vi "Controller Error Handling Loop.vi"(7 "Sync Objects":T1, 8 "error in (no error)":errorcluster, 11 "FOFB Configuration":T4={"FOFB Parameters"={"Network"={"FOFB Controller IP"="", "LNLS Control Network IP"="", "LNLS Control Network Power Supplies TCP Port"=0, "LNLS Control Network FOFB Configuration TCP Port"=0, "LNLS Control Network BPMs TCP Port"=0, "Monitoring Data TCP Port"=0, "Fast Archiver TCP Port"=0, "Fast Command TCP Port"=0, "TCP Listening Timeout"=0}, "Fast Acquisition"={"Sampling Period"=0, "Data Buffer Size"=0, "Monitoring Period"=0}, "Acquisition Network"=[], "Actuation Network"=[]}, "Number of Acquisition Chassis"=0, "Number of Actuation Chassis"=0, "Number of BPM Readings"=0, "BPM Reading Names"=[], "Selected BPM Readings"=[0, 1, 2, 3, 4, 5, 6, 7, 8, 9, 10, 11, 12, 13, 14, 15, 16, 17, 18, 19, 20, 21, 22, 23, 24, 25, 26, 27, 28, 29, 30, 31, 32, 33, 34, 35, 36, 37, 38, 39, 40, 41, 42, 43, 44, 45, 46, 47, 48, 49], "Number of Correctors"=0, "Corrector Names"=[], "Selected Correctors"=[0, 1, 2, 3, 4, 5, 6, 7, 8, 9, 10, 11, 12, 13, 14, 15, 16, 17, 18, 19, 20, 21, 22, 23, 24, 25, 26, 27, 28, 29, 30, 31, 32, 33, 34, 35, 36, 37, 38, 39, 40, 41, 42, 43, 44, 45, 46, 47, 48, 49], "Response Matrix"=[], "Reference Orbit"=[], "Correction Matrix"=[], "FPGA Filter Sets"=[], "Acquisition Chassis Names"=[], "Actuation Chassis Names"=[], "Acquisition Variables"=[], "Actuation Variables"=[], "PS Matrix Mapping"=[], "Inverse PS Matrix Mapping"=[], "BPM Matrix Mapping"=[], "Inverse BPM Matrix Mapping"=[], "BPM Planes"=[], "Corrector Planes"=[]}) -> (0 "error out":errorcluster)   [LabVIEW 2011, in "Controller VIs.lvlib"]
uses:
  Controller VIs.lvlib
  Types Definitions/Type FOFB Configuration.ctl
  Types Definitions/Type FOFB Parameters.ctl
  Types Definitions/Type Network Configuration.ctl
  Types Definitions/Type FA Configuration.ctl
  Types Definitions/Type Acquisition Network Configuration.ctl
  Types Definitions/Type Actuation Network Configuration.ctl
  Types Definitions/Type Synchronization Objects.ctl
  Types Definitions/Type Blocking Synchronization Objects.ctl
  Types Definitions/Type Monitoring Data.ctl
  Types Definitions/Type Operation Mode State.ctl
  Types Definitions/Type Diagnostics Data.ctl
  Types Definitions/Type CPU Loads Array.ctl
  Types Definitions/Type CPU Loads.ctl
  Types Definitions/Type Non-blocking Synchronization Objects.ctl
  Types Definitions/Type FOFB Variables.ctl
  Types Definitions/Type Actuation State.ctl
  <vilib>/Platform/TimedLoop/XDataNode/timing_clust.ctl
  <vilib>/Platform/TimedLoop/XDataNode/nitl_modes.ctl
  <vilib>/Platform/TimedLoop/XDataNode/wakeup.ctl
  <vilib>/Platform/TimedLoop/XDataNode/XDataNode.xnode
  <vilib>/Platform/TimedLoop/XDataNode/XDNodeRunTimeDep.lvlib
  Type Definitions.lvlib
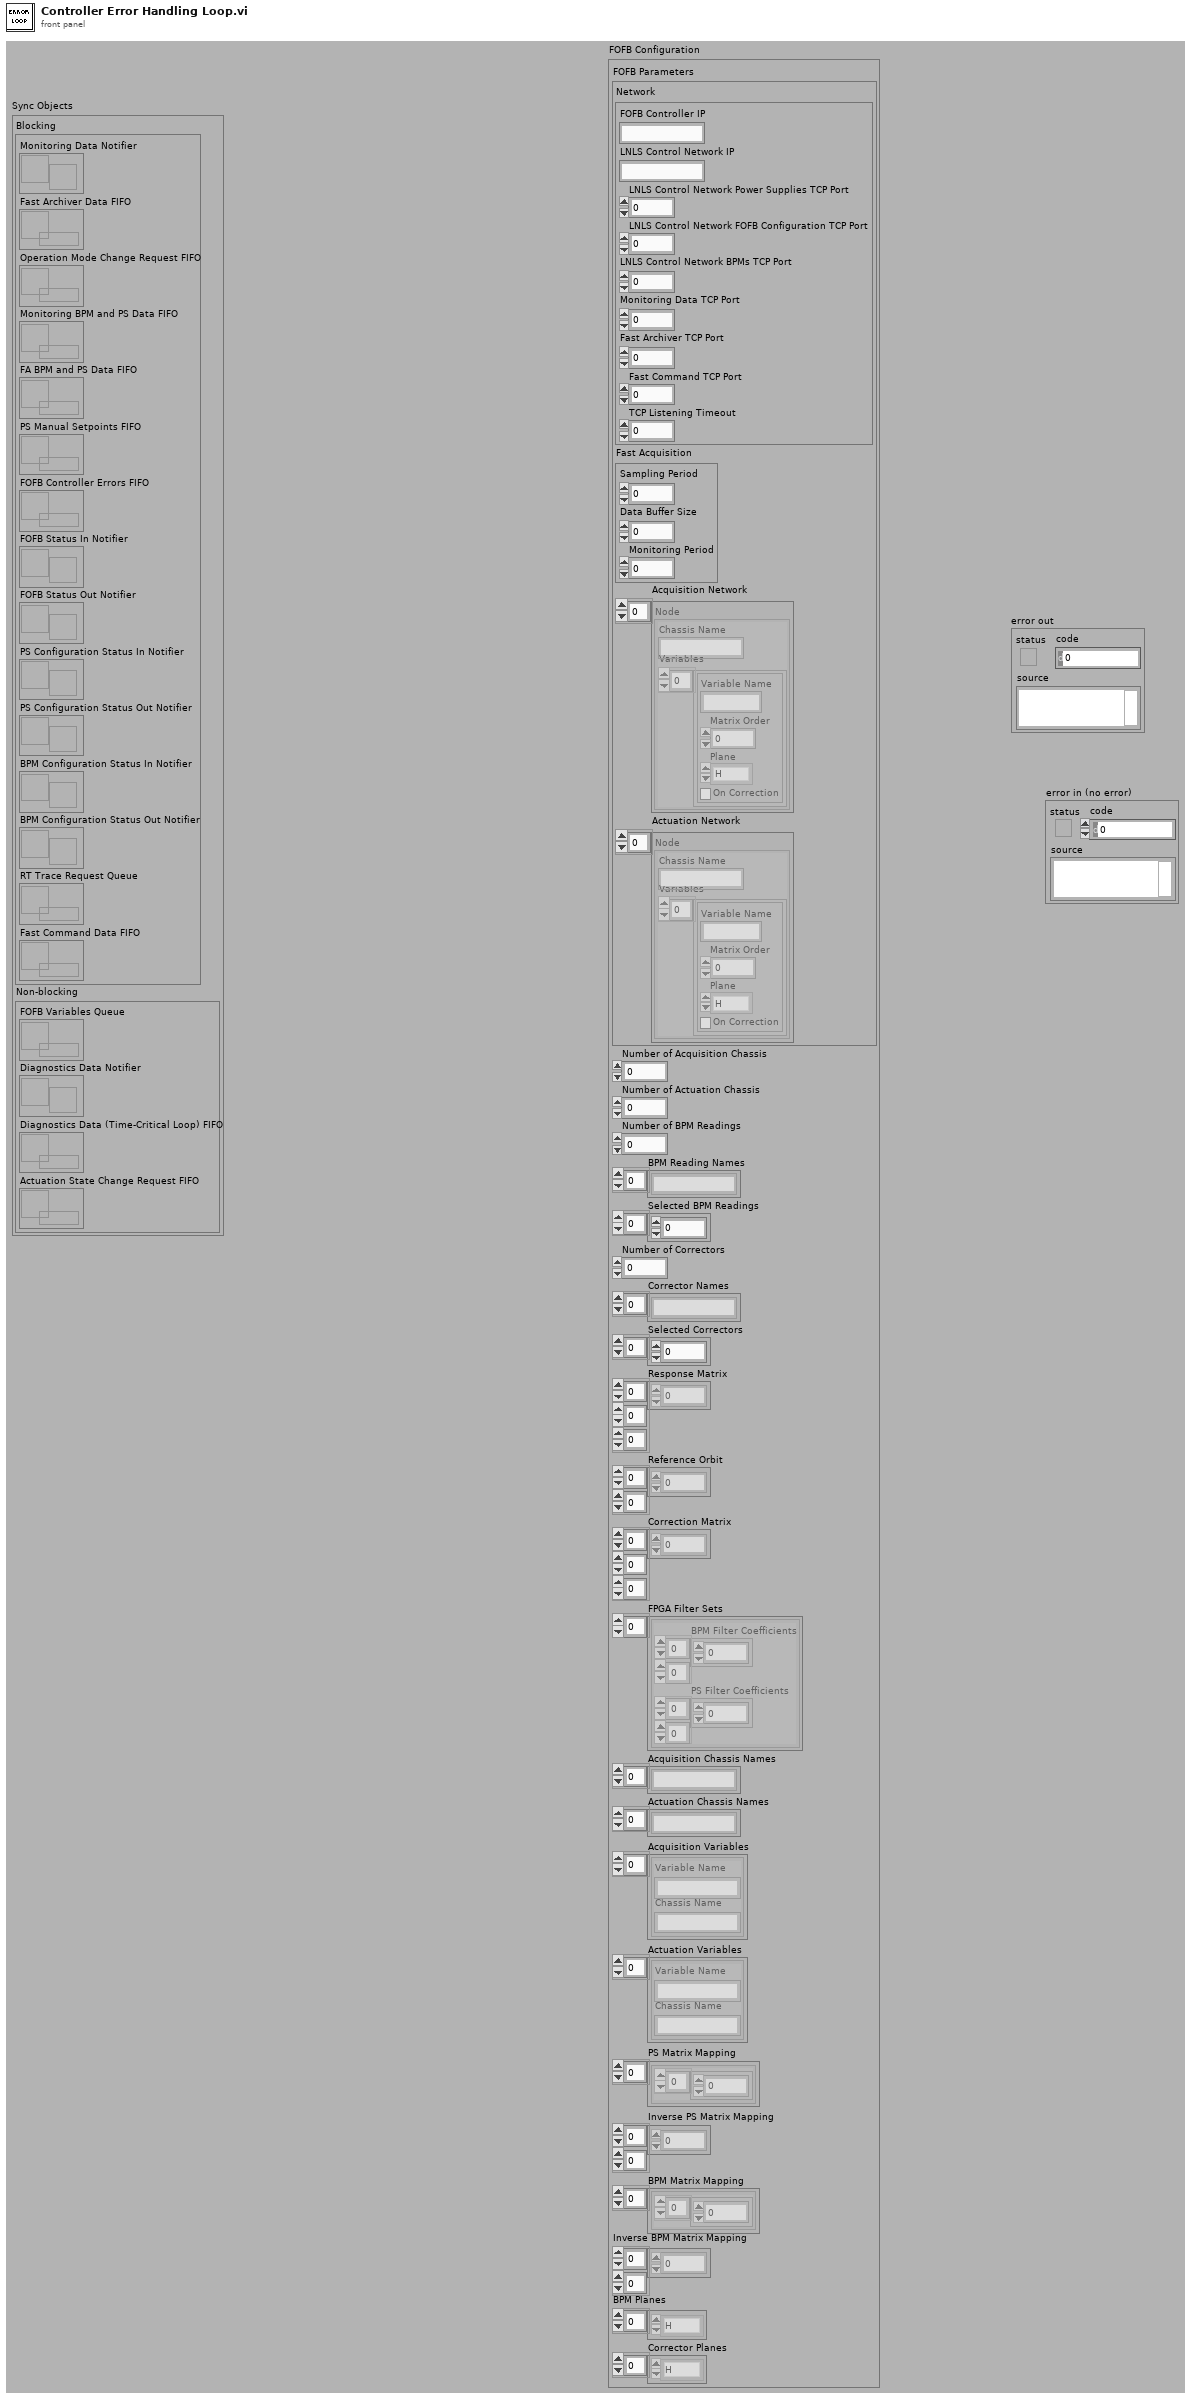
[diagram p1: front panel]
types:
  T1 = typedef "Type Definitions.lvlib/Type Synchronization Objects.ctl" = cluster{"Blocking":T2, "Non-blocking":T3}
  T2 = typedef "Type Definitions.lvlib/Type Blocking Synchronization Objects.ctl" = cluster{"Monitoring Data Notifier":refnum<notifier>, "Fast Archiver Data FIFO":refnum<queue>, "Operation Mode Change Request FIFO":refnum<k33>, "Monitoring BPM and PS Data FIFO":refnum<k33>, "FA BPM and PS Data FIFO":refnum<k33>, "PS Manual Setpoints FIFO":refnum<k33>, "FOFB Controller Errors FIFO ":refnum<k33>, "FOFB Status In Notifier":refnum<notifier>, "FOFB Status Out Notifier":refnum<notifier>, "PS Configuration Status In Notifier":refnum<notifier>, "PS Configuration Status Out Notifier":refnum<notifier>, "BPM Configuration Status In Notifier":refnum<notifier>, "BPM Configuration Status Out Notifier":refnum<notifier>, "RT Trace Request Queue":refnum<queue>, "Fast Command Data FIFO":refnum<k33>}
  T3 = typedef "Type Definitions.lvlib/Type Non-blocking Synchronization Objects.ctl" = cluster{"FOFB Variables Queue":refnum<queue>, "Diagnostics Data Notifier":refnum<notifier>, "Diagnostics Data (Time-Critical Loop) FIFO":refnum<k33>, "Actuation State Change Request FIFO":refnum<k33>}
  T4 = typedef "Type Definitions.lvlib/Type FOFB Configuration.ctl" = cluster{"FOFB Parameters":T5, "Number of Acquisition Chassis":i32, "Number of Actuation Chassis":i32, "Number of BPM Readings":i32, "BPM Reading Names":string[], "Selected BPM Readings":u32[], "Number of Correctors":i32, "Corrector Names":string[], "Selected Correctors":u32[], "Response Matrix":dbl[][][], "Reference Orbit":dbl[][], "Correction Matrix":dbl[][][], "FPGA Filter Sets":cluster{"BPM Filter Coefficients":dbl[][], "PS Filter Coefficients":dbl[][]}[], "Acquisition Chassis Names":string[], "Actuation Chassis Names":string[], "Acquisition Variables":cluster{"Variable Name":string, "Chassis Name":string}[], "Actuation Variables":cluster{"Variable Name":string, "Chassis Name":string}[], "PS Matrix Mapping":cluster{u32[]}[], "Inverse PS Matrix Mapping":u32[][], "BPM Matrix Mapping":cluster{u32[]}[], "Inverse BPM Matrix Mapping":u32[][], "BPM Planes":enum8{"H", "V"}[], "Corrector Planes":enum8{"H", "V"}[]}
  T5 = typedef "Type Definitions.lvlib/Type FOFB Parameters.ctl" = cluster{"Network":T6, "Fast Acquisition":T7, "Acquisition Network":T8, "Actuation Network":T9}
  T6 = typedef "Type Definitions.lvlib/Type Network Configuration.ctl" = cluster{"FOFB Controller IP":string, "LNLS Control Network IP":string, "LNLS Control Network Power Supplies TCP Port":u16, "LNLS Control Network FOFB Configuration TCP Port":u16, "LNLS Control Network BPMs TCP Port":u16, "Monitoring Data TCP Port":u16, "Fast Archiver TCP Port":u16, "Fast Command TCP Port":u16, "TCP Listening Timeout":i32}
  T7 = typedef "Type Definitions.lvlib/Type FA Configuration.ctl" = cluster{"Sampling Period":u32, "Data Buffer Size":u32, "Monitoring Period":u32}
  T8 = typedef "Type Definitions.lvlib/Type Acquisition Network Configuration.ctl" = cluster{"Chassis Name":string, "Variables":cluster{"Variable Name":string, "Matrix Order":u32, "Plane":enum8{"H", "V"}, "On Correction":bool}[]}[]
  T9 = typedef "Type Definitions.lvlib/Type Actuation Network Configuration.ctl" = cluster{"Chassis Name":string, "Variables":cluster{"Variable Name":string, "Matrix Order":u32, "Plane":enum8{"H", "V"}, "On Correction":bool}[]}[]
  T10 = typedef "XDNodeRunTimeDep.lvlib/timing_clust.ctl" = cluster{"Expected End [f-1]":u64, "Actual End [f-1]":u64, "Finished Late? [f-1]":bool, "Expected End [i-1]":u64, "Actual End [i-1]":u64, "Finished Late? [i-1]":bool, "Expected Start [i]":u64, "Actual Start [i]":u64, "Expected Start [f]":u64, "Actual Start [f]":u64, "Source Name":string, "Structure Name":string, "Period":i64, "Deadline":i64, "Offset":i64, "Start":i64, "Priority":i32, "Timeout":i32, "Mode":T11, "Wakeup Reason":T12, "Error":errorcluster, "Source Type":string, "Secondary Source Type":string, "Global End Time":u64, "Global Start Time":u64, "Frame Duration":u64, "Iteration Duration":u64, "Assigned CPU":i32, "I/O Scan Engine Mode":u32}
  T11 = typedef "XDNodeRunTimeDep.lvlib/nitl_modes.ctl" = enum32{"No Change", "Process missed periods, maintain original phase", "Discard missed periods, maintain original phase", "Process missed periods, ignore original phase", "Discard missed periods, ignore original phase"}
  T12 = typedef "XDNodeRunTimeDep.lvlib/wakeup.ctl" = enum32{"Normal", "Aborted", "Asynchronous wakeup", "Timing source error", "Timed loop error", "Timeout"}
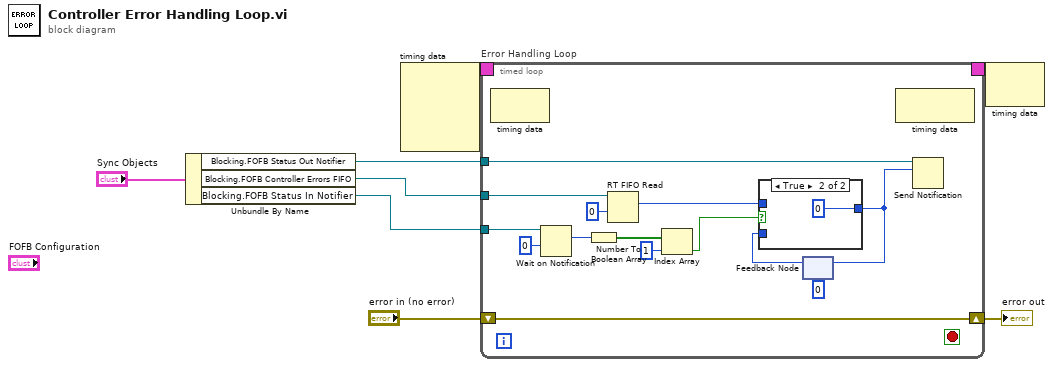
[diagram p0: block diagram]
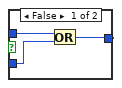
[diagram p2: hidden frame]
diagram:
  n1 = Unbundle By Name("Sync Objects") -> ("Blocking.FOFB Status Out Notifier"=w4:refnum<notifier>, "Blocking.FOFB Controller Errors FIFO"=w2:refnum<k33>, "Blocking.FOFB Status In Notifier"=w5:refnum<notifier>)
  n2 = node-c288() -> (w7:T10)  [unwired: 4 in]
  n3 = timed-loop "Error Handling Loop" {
    shift-right: [w9] -> w1
    shift-left: "error in (no error)" -> [w9]
    tunnel: w2 -> [w22]
    timing: w7 -> [_]
    timing-out: [_] -> w6
    tunnel: w5 -> [w21]
    tunnel: w4 -> [w20]
    stop <- _ stop-if-true
    n4 = node-c288() -> ()  [unwired: 1 in, 1 out]
    n5 = Wait on Notification(notifier=w21, timeout in ms (-1)=0) -> (notification=w11:u16)  [unwired: 2 in, 3 out]
    n6 = Number To Boolean Array(number=w11) -> (Boolean array=w16:bool[])
    n7 = RT FIFO Read(0:w22, 2:0 ("timeout in ms (0)")) -> (9:w19:u16)  [unwired: 2 in, 4 out]
    n8 = Index Array(array=w16, index=1) -> (element=w15:bool)
    n9 = feedback #1(u16 0 ("Controller Error Status")) -> (w17:u16)
    n10 = case shown="True" w15 {
      tunnel: [w23 u16 0 ("Controller Error Status")] -> w13
      tunnel: w19 -> [w25 _]
      tunnel: w17 -> [w24 _]
      frame False {
        n11 = Or(x=w25, y=w24) -> (x .or. y?=w23:u16)
      }
      frame True {
      }
    }
    n12 = feedback-in #1(w13) -> ()
    n13 = node-c288() -> ()  [unwired: 1 in, 1 out]
    n14 = Send Notification(notification=w13, notifier=w20) -> ()  [unwired: 1 in, 2 out]
  }
  "error out" <- w1
  n15 = node-c288(w6) -> ()  [unwired: 1 out]
